vi "g_Stop.vi"() -> ()   [LabVIEW 2014]
panel:
  in  "TestProcSTOP":bool
  in  "STOP":bool
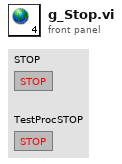
[diagram p1: front panel]
diagram:
